vi "Datasheet Get PIM Result.vi"(6 "Run Information":T1, 8 "DIRECTION":string, 9 "UNITS":string, 11 "PARAMETER":string) -> (3 "Table item":string)   [LabVIEW 2011]
uses:
  TDMS/TDMS Run.ctl
  TDMS/TDMS Channel (Sxx).ctl
  database/Fields/Field Record.ctl
  database/Fields/Field DataTypes.ctl
  database/Fields/Field NextItem.ctl
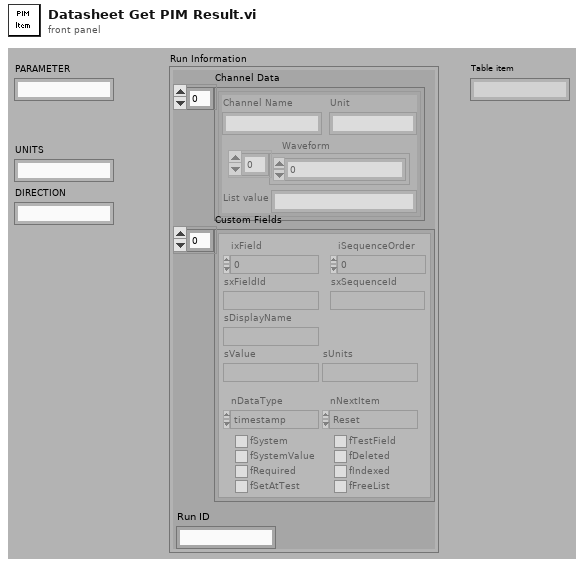
[diagram p1: front panel]
types:
  T1 = typedef "TDMS Run.ctl" = cluster{"Channel Data":T2[], "Custom Fields":T3[], "Run ID":string}
  T2 = typedef "TDMS Channel (Sxx).ctl" = cluster{"Channel Name":string, "Waveform":dbl[], "Unit":string, "List value":string}
  T3 = typedef "Field Record.ctl" = cluster{"ixField":i32, "iSequenceOrder":i32, "sxFieldId":string, "sxSequenceId":string, "sDisplayName":string, "sValue":string, "sUnits":string, "nDataType":T4, "nNextItem":T5, "fSystem":bool, "fSystemValue":bool, "fRequired":bool, "fSetAtTest":bool, "fTestField":bool, "fDeleted":bool, "fIndexed":bool, "fFreeList":bool}
  T4 = typedef "Field DataTypes.ctl" = enum32{"text", "numeric", "list", "timestamp", "boolean"}
  T5 = typedef "Field NextItem.ctl" = enum32{"Reset", "Retain", "Auto-Increment"}
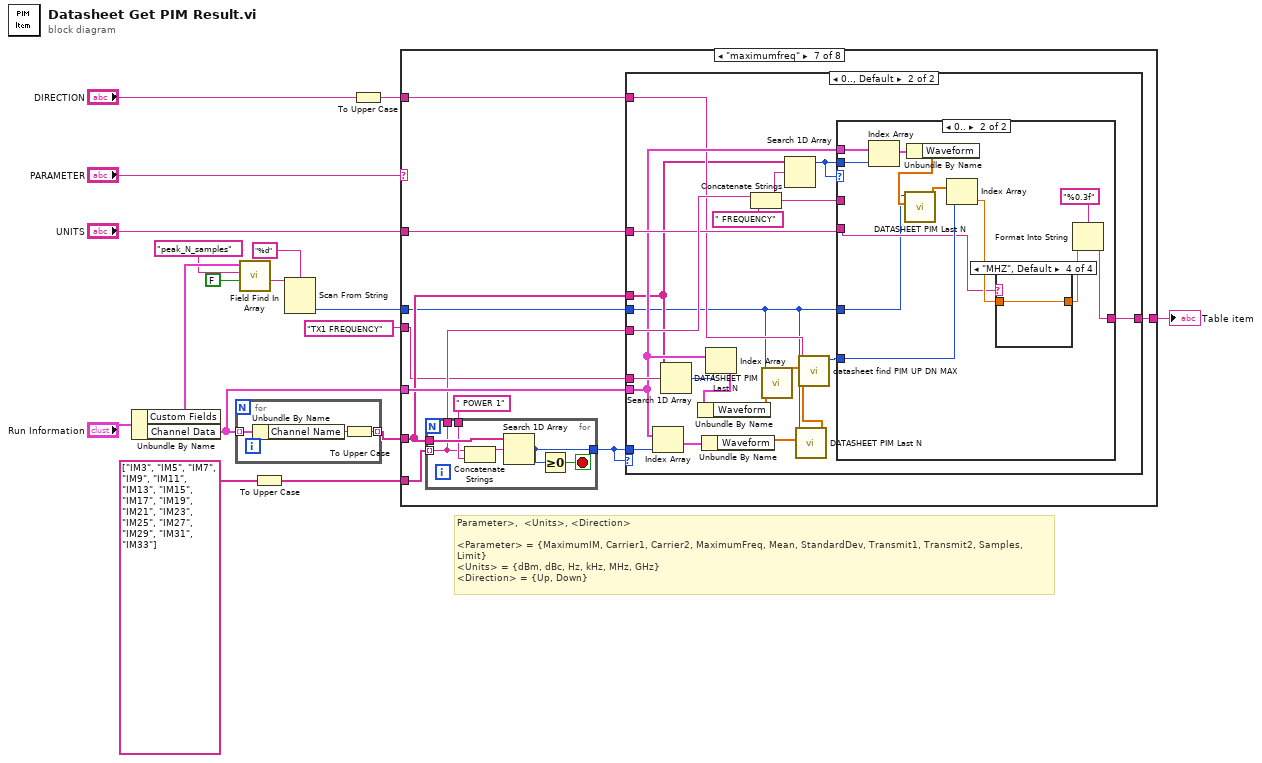
[diagram p0: block diagram]
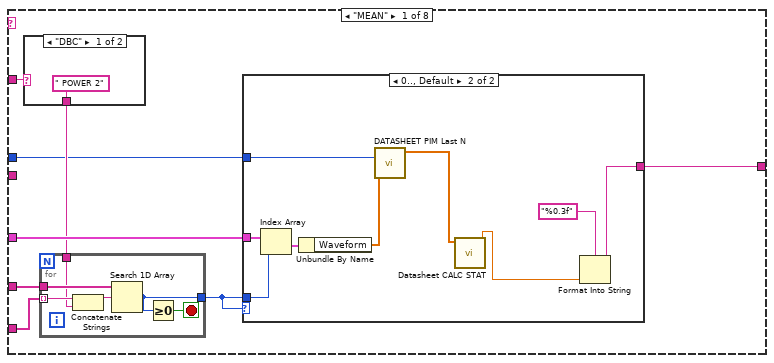
[diagram p2: hidden frame]
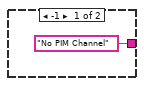
[diagram p3: hidden frame]
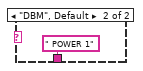
[diagram p4: hidden frame]
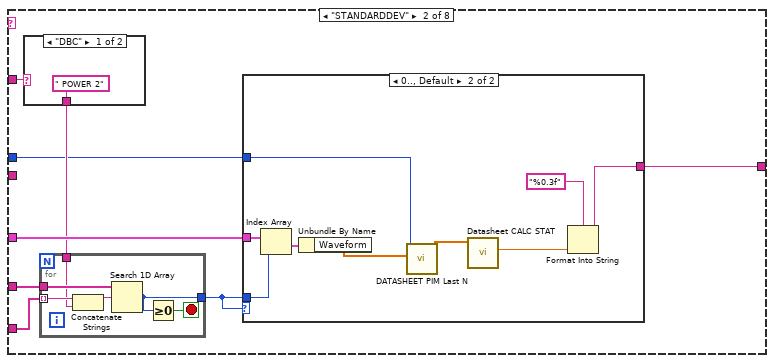
[diagram p5: hidden frame]
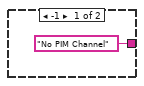
[diagram p6: hidden frame]
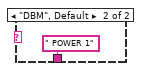
[diagram p7: hidden frame]
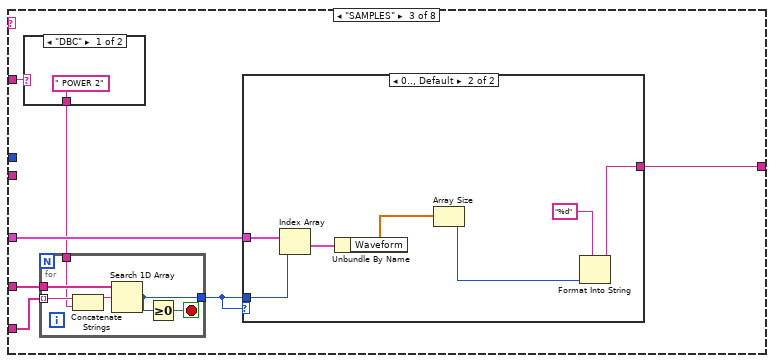
[diagram p8: hidden frame]
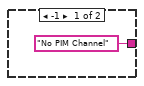
[diagram p9: hidden frame]
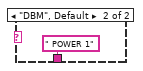
[diagram p10: hidden frame]
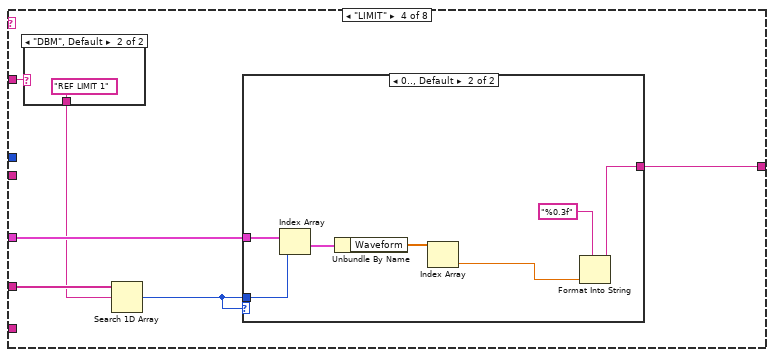
[diagram p11: hidden frame]
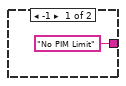
[diagram p12: hidden frame]
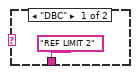
[diagram p13: hidden frame]
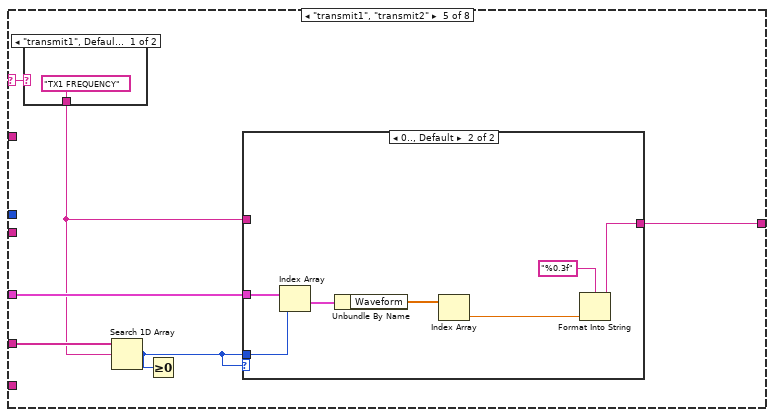
[diagram p14: hidden frame]
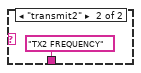
[diagram p15: hidden frame]
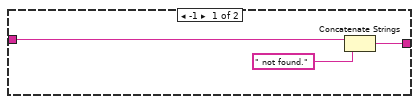
[diagram p16: hidden frame]
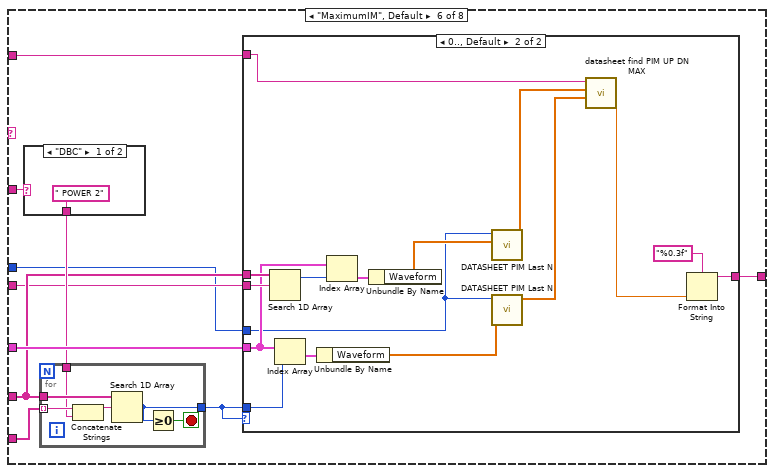
[diagram p17: hidden frame]
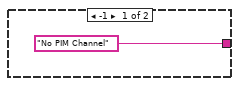
[diagram p18: hidden frame]
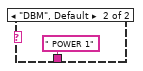
[diagram p19: hidden frame]
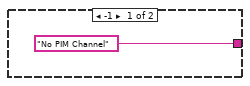
[diagram p20: hidden frame]
diagram:
  # "Parameter>,  <Units>, <Direction>\n\n<Parameter> = {MaximumIM, Carrier1, Carrier2, MaximumFreq, Mean, StandardDev, Transmit1, Transmit2, Samples, Limit}\n<Units> = {dBm, dBc, Hz, kHz, MHz, GHz}\n<Direction> = {Up, Down}"
  n1 = Unbundle By Name("Run Information") -> ("Custom Fields"=w6:T3[], "Channel Data"=w16:T2[])
  n2 = for {
    tunnel: w16 -> [w20] mode=indexing
    tunnel: [w18] -> w13 mode=indexing
    n3 = Unbundle By Name(w20) -> ("Channel Name"=w19:string)
    n4 = To Upper Case(1:w19) -> (0:w18:string)
  }
  n5 = call "Field Find In Array.vi"("by DisplayName? (f, by FieldId)"=FALSE, "FieldID or Display Name(\"\")"="peak_N_samples", "Field Array"=w6) -> ("sValue"=w3:string)  [unwired: 8 out]
  n6 = To Upper Case(1:string[] ["IM3", "IM5", "IM7", "IM9", "IM11", "IM13", "IM15", "IM17", "IM19", "IM21", "IM23", "IM25", "IM27", "IM29", "IM31", "IM33"]) -> (0:w7:string[])
  n7 = Scan From String(format string="%d", input string=w3) -> (output 1=w2:i32)  [unwired: 2 in, 4 out]
  n8 = To Upper Case(1:"DIRECTION") -> (0:w9:string)
  n9 = case shown="\"maximumfreq\"" "PARAMETER" {
    selector: "PARAMETER" -> [_ _ _ _ w113 _ _ w230]
    tunnel: w16 -> [w28 w54 w79 w101 w117 w139 w175 w239]
    tunnel: [w27 w53 w78 w100 w116 w138 w174 w238] -> w11
    tunnel: "UNITS" -> [w26 w52 w77 w99 _ w137 w169 w233]
    tunnel: w13 -> [w25 w51 w76 w98 w115 w132 w168 w234]
    tunnel: w7 -> [w24 w50 w75 _ _ w136 w173 w237]
    tunnel: w9 -> [_ _ _ _ _ w133 w166 w231]
    tunnel: "TX1 FREQUENCY" -> [_ _ _ _ _ w131 w167 w232]
    tunnel: w2 -> [w21 w47 _ _ _ w130 w165 w228]
    frame "MEAN" {
      n10 = case shown="\"DBC\"" w26 {
        tunnel: [" POWER 2" " POWER 1"] -> w23
        frame "DBC" {
        }
        frame "DBM", Default {
        }
      }
      n11 = for {
        tunnel: w25 -> [w44]
        tunnel: w24 -> [w43] mode=indexing
        tunnel: [w40] -> w22
        tunnel: w23 -> [w39]
        stop <- w41 stop-if-true
        n12 = Concatenate Strings(w43, w39) -> (w42:string)
        n13 = Search 1D Array(1D array=w44, element=w42) -> (index of element=w40:i32)  [unwired: 1 out]
        n14 = Greater Or Equal To 0?(x=w40) -> (x >= 0?=w41:bool)
      }
      n15 = case shown="0.., Default" w22 {
        tunnel: w28 -> [_ w37]
        tunnel: ["No PIM Channel" w35] -> w27
        tunnel: w22 -> [_ w36]
        tunnel: w21 -> [_ w30]
        frame -1 {
        }
        frame 0.., Default {
          n16 = Index Array(array=w37, index=w36) -> (element=w38:T2)
          n17 = Unbundle By Name(w38) -> ("Waveform"=w31:dbl[])
          n18 = call "DATASHEET PIM Last N.vi"("full waveform"=w31, "n points"=w30) -> ("last n pnts waveform"=w32:dbl[])  [unwired: 9 out]
          n19 = call "Datasheet CALC STAT.vi"("Channel Data"=w32) -> ("Mean"=w34:dbl)  [unwired: 10 out]
          n20 = Format Into String(format string="%0.3f", w34) -> (resulting string=w35:string)  [unwired: 2 in, 1 out]
        }
      }
    }
    frame "STANDARDDEV" {
      n21 = case shown="\"DBC\"" w52 {
        tunnel: [" POWER 2" " POWER 1"] -> w49
        frame "DBC" {
        }
        frame "DBM", Default {
        }
      }
      n22 = for {
        tunnel: w51 -> [w70]
        tunnel: w50 -> [w69] mode=indexing
        tunnel: [w66] -> w48
        tunnel: w49 -> [w65]
        stop <- w67 stop-if-true
        n23 = Concatenate Strings(w69, w65) -> (w68:string)
        n24 = Search 1D Array(1D array=w70, element=w68) -> (index of element=w66:i32)  [unwired: 1 out]
        n25 = Greater Or Equal To 0?(x=w66) -> (x >= 0?=w67:bool)
      }
      n26 = case shown="0.., Default" w48 {
        tunnel: w54 -> [_ w63]
        tunnel: ["No PIM Channel" w61] -> w53
        tunnel: w48 -> [_ w62]
        tunnel: w47 -> [_ w58]
        frame -1 {
        }
        frame 0.., Default {
          n27 = Index Array(array=w63, index=w62) -> (element=w64:T2)
          n28 = Unbundle By Name(w64) -> ("Waveform"=w57:dbl[])
          n29 = call "DATASHEET PIM Last N.vi"("full waveform"=w57, "n points"=w58) -> ("last n pnts waveform"=w56:dbl[])  [unwired: 9 out]
          n30 = call "Datasheet CALC STAT.vi"("Channel Data"=w56) -> ("Standard Deviation"=w60:dbl)  [unwired: 10 out]
          n31 = Format Into String(format string="%0.3f", w60) -> (resulting string=w61:string)  [unwired: 2 in, 1 out]
        }
      }
    }
    frame "SAMPLES" {
      n32 = case shown="\"DBC\"" w77 {
        tunnel: [" POWER 2" " POWER 1"] -> w74
        frame "DBC" {
        }
        frame "DBM", Default {
        }
      }
      n33 = for {
        tunnel: w76 -> [w93]
        tunnel: w75 -> [w92] mode=indexing
        tunnel: [w89] -> w73
        tunnel: w74 -> [w88]
        stop <- w90 stop-if-true
        n34 = Concatenate Strings(w92, w88) -> (w91:string)
        n35 = Search 1D Array(1D array=w93, element=w91) -> (index of element=w89:i32)  [unwired: 1 out]
        n36 = Greater Or Equal To 0?(x=w89) -> (x >= 0?=w90:bool)
      }
      n37 = case shown="0.., Default" w73 {
        tunnel: w79 -> [_ w86]
        tunnel: ["No PIM Channel" w84] -> w78
        tunnel: w73 -> [_ w85]
        frame -1 {
        }
        frame 0.., Default {
          n38 = Index Array(array=w86, index=w85) -> (element=w87:T2)
          n39 = Unbundle By Name(w87) -> ("Waveform"=w83:dbl[])
          n40 = Array Size(array=w83) -> (size(s)=w81:i32)
          n41 = Format Into String(format string="%d", w81) -> (resulting string=w84:string)  [unwired: 2 in, 1 out]
        }
      }
    }
    frame "LIMIT" {
      n42 = case shown="\"DBM\", Default" w99 {
        tunnel: ["REF LIMIT 2" "REF LIMIT 1"] -> w97
        frame "DBC" {
        }
        frame "DBM", Default {
        }
      }
      n43 = Search 1D Array(1D array=w98, element=w97) -> (index of element=w96:i32)  [unwired: 1 out]
      n44 = case shown="0.., Default" w96 {
        tunnel: w101 -> [_ w108]
        tunnel: ["No PIM Limit" w106] -> w100
        tunnel: w96 -> [_ w107]
        frame -1 {
        }
        frame 0.., Default {
          n45 = Index Array(array=w108, index=w107) -> (element=w109:T2)
          n46 = Unbundle By Name(w109) -> ("Waveform"=w104:dbl[])
          n47 = Index Array(array=w104) -> (element=w103:dbl)  [unwired: 1 in]
          n48 = Format Into String(format string="%0.3f", w103) -> (resulting string=w106:string)  [unwired: 2 in, 1 out]
        }
      }
    }
    frame "transmit1", "transmit2" {
      n49 = case shown="\"transmit1\", Default" w113 {
        tunnel: ["TX1 FREQUENCY" "TX2 FREQUENCY"] -> w112
        frame "transmit1", Default {
        }
        frame "transmit2" {
        }
      }
      n50 = Search 1D Array(1D array=w115, element=w112) -> (index of element=w114:i32)  [unwired: 1 out]
      n51 = Greater Or Equal To 0?(x=w114) -> ()  [unwired: 1 out]
      n52 = case shown="0.., Default" w114 {
        tunnel: w117 -> [_ w128]
        tunnel: [w121 w126] -> w116
        tunnel: w114 -> [_ w127]
        tunnel: w112 -> [w120 _]
        frame -1 {
          n53 = Concatenate Strings(w120, " not found.") -> (w121:string)
        }
        frame 0.., Default {
          n54 = Index Array(array=w128, index=w127) -> (element=w129:T2)
          n55 = Unbundle By Name(w129) -> ("Waveform"=w125:dbl[])
          n56 = Index Array(array=w125) -> (element=w124:dbl)  [unwired: 1 in]
          n57 = Format Into String(format string="%0.3f", w124) -> (resulting string=w126:string)  [unwired: 2 in, 1 out]
        }
      }
    }
    frame "MaximumIM", Default {
      n58 = case shown="\"DBC\"" w137 {
        tunnel: [" POWER 2" " POWER 1"] -> w135
        frame "DBC" {
        }
        frame "DBM", Default {
        }
      }
      n59 = for {
        tunnel: w132 -> [w162]
        tunnel: w136 -> [w161] mode=indexing
        tunnel: [w158] -> w134
        tunnel: w135 -> [w157]
        stop <- w159 stop-if-true
        n60 = Concatenate Strings(w161, w157) -> (w160:string)
        n61 = Search 1D Array(1D array=w162, element=w160) -> (index of element=w158:i32)  [unwired: 1 out]
        n62 = Greater Or Equal To 0?(x=w158) -> (x >= 0?=w159:bool)
      }
      n63 = case shown="0.., Default" w134 {
        tunnel: w139 -> [_ w150]
        tunnel: ["No PIM Channel" w154] -> w138
        tunnel: w134 -> [_ w155]
        tunnel: w133 -> [_ w148]
        tunnel: w132 -> [_ w153]
        tunnel: w131 -> [_ w152]
        tunnel: w130 -> [_ w141]
        frame -1 {
        }
        frame 0.., Default {
          n64 = Search 1D Array(1D array=w153, element=w152) -> (index of element=w151:i32)  [unwired: 1 out]
          n65 = Index Array(array=w150, index=w155) -> (element=w156:T2)
          n66 = Unbundle By Name(w156) -> ("Waveform"=w143:dbl[])
          n67 = Index Array(array=w150, index=w151) -> (element=w149:T2)
          n68 = Unbundle By Name(w149) -> ("Waveform"=w145:dbl[])
          n69 = call "DATASHEET PIM Last N.vi"("full waveform"=w145, "n points"=w141) -> ("last n pnts waveform"=w144:dbl[])  [unwired: 9 out]
          n70 = call "DATASHEET PIM Last N.vi"("full waveform"=w143, "n points"=w141) -> ("last n pnts waveform"=w142:dbl[])  [unwired: 9 out]
          n71 = call "datasheet find PIM UP DN MAX.vi"("im power waveform"=w142, "tx1 frequency"=w144, "direction"=w148) -> ("max"=w146:dbl)  [unwired: 8 out]
          n72 = Format Into String(format string="%0.3f", w146) -> (resulting string=w154:string)  [unwired: 2 in, 1 out]
        }
      }
    }
    frame "maximumfreq" {
      n73 = for {
        tunnel: w168 -> [w227]
        tunnel: w173 -> [w222] mode=indexing
        tunnel: [w224] -> w171
        tunnel: " POWER 1" -> [w223]
        tunnel: [w222] -> w170
        stop <- w225 stop-if-true
        n74 = Concatenate Strings(w222, w223) -> (w226:string)
        n75 = Search 1D Array(1D array=w227, element=w226) -> (index of element=w224:i32)  [unwired: 1 out]
        n76 = Greater Or Equal To 0?(x=w224) -> (x >= 0?=w225:bool)
      }
      n77 = case shown="0.., Default" w171 {
        tunnel: w175 -> [_ w186]
        tunnel: ["No PIM Channel" w194] -> w174
        tunnel: w171 -> [_ w195]
        tunnel: w170 -> [_ w193]
        tunnel: w168 -> [_ w182]
        tunnel: w169 -> [_ w189]
        tunnel: w167 -> [_ w187]
        tunnel: w166 -> [_ w183]
        tunnel: w165 -> [_ w177]
        frame -1 {
        }
        frame 0.., Default {
          n78 = Index Array(array=w186, index=w195) -> (element=w196:T2)
          n79 = Search 1D Array(1D array=w182, element=w187) -> (index of element=w185:i32)  [unwired: 1 out]
          n80 = Unbundle By Name(w196) -> ("Waveform"=w181:dbl[])
          n81 = Index Array(array=w186, index=w185) -> (element=w184:T2)
          n82 = Unbundle By Name(w184) -> ("Waveform"=w180:dbl[])
          n83 = Concatenate Strings(w193, " FREQUENCY") -> (w190:string)
          n84 = call "DATASHEET PIM Last N.vi"("full waveform"=w180, "n points"=w177) -> ("last n pnts waveform"=w179:dbl[])  [unwired: 9 out]
          n85 = Search 1D Array(1D array=w182, element=w190) -> (index of element=w191:i32)  [unwired: 1 out]
          n86 = call "DATASHEET PIM Last N.vi"("full waveform"=w181, "n points"=w177) -> ("last n pnts waveform"=w178:dbl[])  [unwired: 9 out]
          n87 = call "datasheet find PIM UP DN MAX.vi"("im power waveform"=w178, "tx1 frequency"=w179, "direction"=w183) -> ("max index"=w188:i32)  [unwired: 8 out]
          n88 = case shown="0.." w191 {
            tunnel: [w198 w211] -> w194
            tunnel: w186 -> [_ w210]
            tunnel: w191 -> [_ w209]
            tunnel: w190 -> [w199 _]
            tunnel: w188 -> [_ w207]
            tunnel: w189 -> [_ w205]
            tunnel: w177 -> [_ w200]
            frame -1, Default {
              n89 = Concatenate Strings(w199, " not found.") -> (w198:string)
            }
            frame 0.. {
              n90 = Index Array(array=w210, index=w209) -> (element=w208:T2)
              n91 = Unbundle By Name(w208) -> ("Waveform"=w201:dbl[])
              n92 = call "DATASHEET PIM Last N.vi"("full waveform"=w201, "n points"=w200) -> ("last n pnts waveform"=w202:dbl[])  [unwired: 9 out]
              n93 = Index Array(array=w202, index=w207) -> (element=w206:dbl)
              n94 = case shown="\"MHZ\", Default" w205 {
                tunnel: w206 -> [w214 w217 w220 w221]
                tunnel: [w213 w216 w219 w221] -> w204
                frame "HZ" {
                  n95 = Multiply(x=w214, y=1000000.0) -> (x*y=w213:dbl)
                }
                frame "KHZ" {
                  n96 = Multiply(x=w217, y=100000.0) -> (x*y=w216:dbl)
                }
                frame "GHZ" {
                  n97 = Divide(x=w220, y=1000.0) -> (x/y=w219:dbl)
                }
                frame "MHZ", Default {
                }
              }
              n98 = Format Into String(format string="%0.3f", w204) -> (resulting string=w211:string)  [unwired: 2 in, 1 out]
            }
          }
        }
      }
    }
    frame "CARRIER1", "CARRIER2" {
      n99 = for {
        tunnel: w234 -> [w291]
        tunnel: w237 -> [w286] mode=indexing
        tunnel: [w288] -> w235
        tunnel: " POWER 1" -> [w287]
        tunnel: [w286] -> _
        stop <- w289 stop-if-true
        n100 = Concatenate Strings(w286, w287) -> (w290:string)
        n101 = Search 1D Array(1D array=w291, element=w290) -> (index of element=w288:i32)  [unwired: 1 out]
        n102 = Greater Or Equal To 0?(x=w288) -> (x >= 0?=w289:bool)
      }
      n103 = case shown="\"CARRIER2\"" w230 {
        tunnel: ["TX1 FREQUENCY" "TX2 FREQUENCY"] -> w229
        frame "CARRIER1", Default {
        }
        frame "CARRIER2" {
        }
      }
      n104 = case shown="0.., Default" w235 {
        tunnel: w239 -> [_ w253]
        tunnel: ["No PIM Channel" w258] -> w238
        tunnel: w235 -> [_ w259]
        tunnel: w234 -> [_ w252]
        tunnel: w233 -> [_ w256]
        tunnel: w232 -> [_ w251]
        tunnel: w231 -> [_ w249]
        tunnel: w229 -> [_ w248]
        tunnel: w228 -> [_ w243]
        frame -1 {
        }
        frame 0.., Default {
          n105 = Index Array(array=w253, index=w259) -> (element=w260:T2)
          n106 = Search 1D Array(1D array=w252, element=w251) -> (index of element=w255:i32)  [unwired: 1 out]
          n107 = Unbundle By Name(w260) -> ("Waveform"=w247:dbl[])
          n108 = Index Array(array=w253, index=w255) -> (element=w254:T2)
          n109 = Unbundle By Name(w254) -> ("Waveform"=w244:dbl[])
          n110 = call "DATASHEET PIM Last N.vi"("full waveform"=w244, "n points"=w243) -> ("last n pnts waveform"=w245:dbl[])  [unwired: 9 out]
          n111 = Search 1D Array(1D array=w252, element=w248) -> (index of element=w257:i32)  [unwired: 1 out]
          n112 = call "DATASHEET PIM Last N.vi"("full waveform"=w247, "n points"=w243) -> ("last n pnts waveform"=w246:dbl[])  [unwired: 9 out]
          n113 = call "datasheet find PIM UP DN MAX.vi"("im power waveform"=w246, "tx1 frequency"=w245, "direction"=w249) -> ("max index"=w250:i32)  [unwired: 8 out]
          n114 = case shown="0.." w257 {
            tunnel: [w262 w275] -> w258
            tunnel: w253 -> [_ w274]
            tunnel: w257 -> [_ w273]
            tunnel: w248 -> [w263 _]
            tunnel: w250 -> [_ w271]
            tunnel: w256 -> [_ w267]
            tunnel: w243 -> [_ w266]
            frame -1, Default {
              n115 = Concatenate Strings(w263, " not found.") -> (w262:string)
            }
            frame 0.. {
              n116 = Index Array(array=w274, index=w273) -> (element=w272:T2)
              n117 = Unbundle By Name(w272) -> ("Waveform"=w264:dbl[])
              n118 = call "DATASHEET PIM Last N.vi"("full waveform"=w264, "n points"=w266) -> ("last n pnts waveform"=w265:dbl[])  [unwired: 9 out]
              n119 = Index Array(array=w265, index=w271) -> (element=w269:dbl)
              n120 = case shown="\"MHZ\", Default" w267 {
                tunnel: w269 -> [w278 w281 w284 w285]
                tunnel: [w277 w280 w283 w285] -> w268
                frame "HZ" {
                  n121 = Multiply(x=w278, y=1000000.0) -> (x*y=w277:dbl)
                }
                frame "KHZ" {
                  n122 = Multiply(x=w281, y=100000.0) -> (x*y=w280:dbl)
                }
                frame "GHZ" {
                  n123 = Divide(x=w284, y=1000.0) -> (x/y=w283:dbl)
                }
                frame "MHZ", Default {
                }
              }
              n124 = Format Into String(format string="%0.3f", w268) -> (resulting string=w275:string)  [unwired: 2 in, 1 out]
            }
          }
        }
      }
    }
  }
  "Table item" <- w11
